vi "测试条件.vi"(11 "TimingControl 输入":refnum<class "TimingControl.lvclass">) -> (2 "簇":cluster{bool, "控制命令":T1, "测量参数":T2}, 3 "TimingControl 输出":refnum<class "TimingControl.lvclass">)   [LabVIEW 2022 SP3, in "TimingControl.lvlib" / "TimingControl.lvclass"]
uses:
  TimingControl.lvclass
  TimingControl.lvclass/TimingControl.ctl
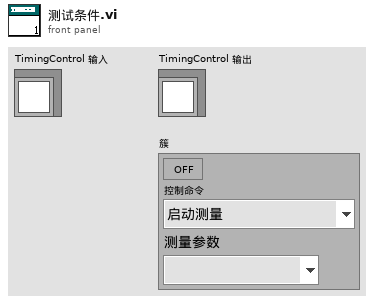
[diagram p1: front panel]
types:
  T1 = typedef "TimingControl.lvlib/TimingControl.lvclass/国标控制命令.ctl" = enum16{"启动测量", "标样核查", "零点核查", "跨度核查", "空白测试", "平行样测试", "加标回收", "空白校准", "标样校准", "初始化（清洗）", "停止测试", "仪器重启", "校时", "模式设置", "测量间隔设置"}
  T2 = typedef "TimingControl.lvlib/TimingControl.lvclass/测量参数.ctl" = u16
  T3 = typedef "TimingControl.lvlib/TimingControl.lvclass/周期模式设置.ctl" = enum16{"不启用", "定点模式", "间隔模式"}
  T4 = typedef "TimingControl.lvlib/TimingControl.lvclass/State Data.ctl" = cluster{"仪器时间":timestamp, "仪器运行状态":bool, "配置文件路径":path, "测量参数":u16, "测试状态":cluster{"启动时间":timestamp, "结束时间":timestamp, "启动次数":i32}, "配置信息":T5}
  T5 = typedef "TimingControl.lvlib/TimingControl.lvclass/配置信息.ctl" = cluster{"每周启动":T6, "每月启动":T7, "周期模式":T3, "测量参数":T2, "定点周期":T8, "间隔启动":T10, "配置时间":timestamp}
  T6 = typedef "TimingControl.lvlib/TimingControl.lvclass/每周启动.ctl" = enum16{"关闭", "周日", "周一", "周二", "周三", "周四", "周五", "周六"}
  T7 = typedef "TimingControl.lvlib/TimingControl.lvclass/每月启动.ctl" = enum16{"关闭", "1号", "2号", "3号", "4号", "5号", "6号", "7号", "8号", "9号", "10号", "11号", "12号", "13号", "14号", "15号", "16号", "17号", "18号", "19号", "20号", "21号", "22号", "23号", "24号", "25号", "26号", "27号", "28号", "29号", "30号", "31号"}
  T8 = typedef "TimingControl.lvlib/TimingControl.lvclass/定点周期设置.ctl" = cluster{"启动命令":T9, "启动命令 2":T9, "启动命令 3":T9, "启动命令 4":T9, "启动命令 5":T9, "启动命令 6":T9, "启动命令 7":T9, "启动命令 8":T9, "启动命令 9":T9, "启动命令 10":T9, "启动命令 11":T9, "启动命令 12":T9, "启动命令 13":T9, "启动命令 14":T9, "启动命令 15":T9, "启动命令 16":T9, "启动命令 17":T9, "启动命令 18":T9, "启动命令 19":T9, "启动命令 20":T9, "启动命令 21":T9, "启动命令 22":T9, "启动命令 23":T9, "启动命令 24":T9}
  T9 = typedef "TimingControl.lvlib/TimingControl.lvclass/启动命令选择.ctl" = enum16{"", "水样测试", "标样核查", "零点核查", "跨度核查", "空白测试", "平行样测试", "加标回收", "空白校准", "标样校准", "初始化(清洗)"}
  T10 = typedef "TimingControl.lvlib/TimingControl.lvclass/间隔启动设置.ctl" = cluster{"启动命令":T9, "启动间隔":dbl, "启动次数":i32}
  T11 = typedef "LVDateTimeRec.ctl" = cluster{"秒数的小数部分":dbl, "秒":i32, "分":i32, "时":i32, "日":i32, "月":i32, "年":i32, "天数（周）":i32, "天数（年）":i32, "DST":i32}
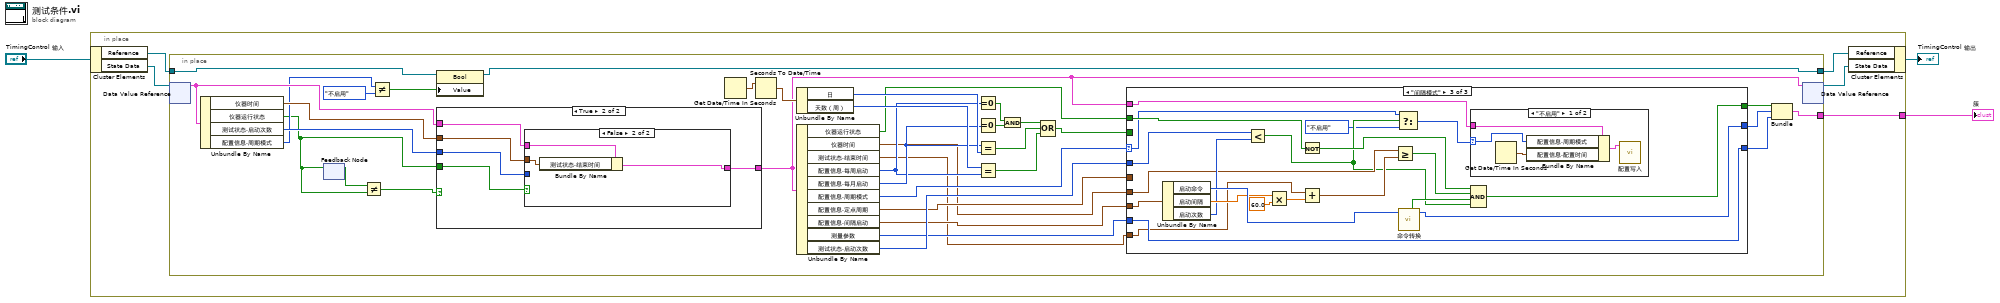
[diagram p0: block diagram]
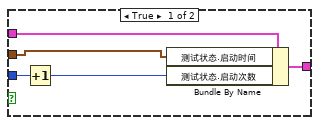
[diagram p3: hidden frame]
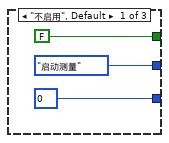
[diagram p4: hidden frame]
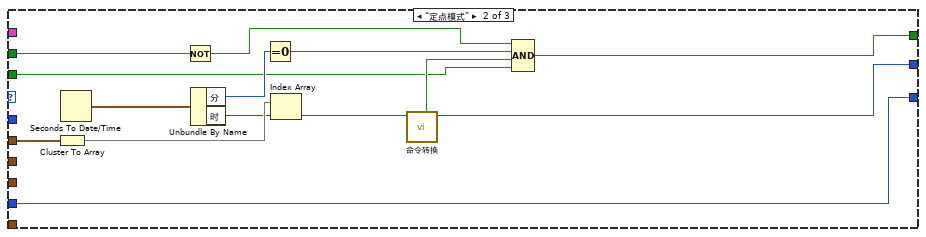
[diagram p5: hidden frame]
diagram:
  n1 = in-place {
    in-place-border: [w8] -> w3
    n2 = in-place-cluster #1("TimingControl 输入") -> ("Reference"=w7:refnum<vi>, "State Data"=w6:refnum<data-value>)
    n3 = in-place {
      in-place-border: w7 -> [w16]
      in-place-border: [w14] -> w8
      in-place-border: [w12] -> w4
      n4 = in-place-dvr #2(w6) -> (w19:T4)  [unwired: 1 out]
      n5 = Unbundle By Name(w19) -> ("仪器时间"=w26:timestamp, "仪器运行状态"=w10:bool, "测试状态.启动次数"=w25:i32, "配置信息.周期模式"=w15:T3)
      n6 = feedback-in #3(w10) -> ()
      n7 = feedback #3() -> (w11:bool)  [unwired: 1 in]
      n8 = Not Equal?(x=w11, y=w10) -> (x != y?=w9:bool)
      n9 = Not Equal?(x=w15, y=周期模式设置."不启用") -> (x != y?=w17:bool)
      n10 = property class="Bool"(reference=w16, "Value"=w17) -> (reference out=w12:refnum<vi>)  [unwired: 1 in, 1 out]
      n11 = case shown="True" w9 {
        tunnel: w26 -> [_ w50]
        tunnel: w25 -> [_ w49]
        tunnel: [w45 w48] -> w13
        tunnel: w19 -> [w45 w47]
        tunnel: w10 -> [_ w46]
        frame False {
        }
        frame True {
          n12 = case shown="False" w46 {
            tunnel: w50 -> [w55 w58]
            tunnel: w49 -> [w53 _]
            tunnel: [w52 w57] -> w48
            tunnel: w47 -> [w51 w56]
            frame True {
              n13 = Increment(x=w53) -> (x+1=w54:i32)
              n14 = Bundle By Name(cluster=w51, "测试状态.启动时间"=w55, "测试状态.启动次数"=w54) -> (w52:T4)
            }
            frame False {
              n15 = Bundle By Name(cluster=w56, "测试状态.结束时间"=w58) -> (w57:T4)
            }
          }
        }
      }
      n16 = Get Date/Time In Seconds() -> (seconds since 1Jan1904=w32:timestamp)
      n17 = Seconds To Date/Time(time stamp (now)=w32) -> (date time rec=w36:T11)  [unwired: 1 in]
      n18 = Unbundle By Name(w36) -> ("日"=w31:i32, "天数（周）"=w35:i32)
      n19 = Unbundle By Name(w13) -> ("仪器运行状态"=w24:bool, "仪器时间"=w21:timestamp, "测试状态.结束时间"=w20:timestamp, "配置信息.每周启动"=w28:T6, "配置信息.每月启动"=w30:T7, "配置信息.周期模式"=w43:T3, "配置信息.定点周期"=w42:T8, "配置信息.间隔启动"=w41:T10, "测量参数"=w40:u16, "测试状态.启动次数"=w44:i32)
      n20 = Equal To 0?(x=w28) -> (x = 0?=w22:bool)
      n21 = Equal To 0?(x=w30) -> (x = 0?=w29:bool)
      n22 = Equal?(x=w30, y=w31) -> (x = y?=w34:bool)
      n23 = Equal?(x=w35, y=w28) -> (x = y?=w33:bool)
      n24 = And(x=w22, y=w29) -> (x .and. y?=w23:bool)
      n25 = Compound Arithmetic op=OR ("复合运算")(w23, w34, w33) -> (w27:bool)
      n26 = case shown="\"间隔模式\"" w43 {
        selector: w43 -> [_ _ w79]
        tunnel: w42 -> [_ w66 _]
        tunnel: w41 -> [_ _ w91]
        tunnel: w40 -> [_ w70 w94]
        tunnel: [国标控制命令."启动测量" ("控制命令") w68 w92] -> w38
        tunnel: [FALSE w71 w95] -> w39
        tunnel: [w59 w70 w94] -> w37
        tunnel: w27 -> [_ w67 _]
        tunnel: w24 -> [_ w62 w84]
        tunnel: w44 -> [_ _ w83]
        tunnel: w20 -> [_ _ w82]
        tunnel: w21 -> [_ _ w81]
        tunnel: w13 -> [_ _ w76]
        frame "不启用", Default {
          w59 = T2 0 items=[""] ("测量参数")
        }
        frame "定点模式" {
          n27 = Cluster To Array(cluster=w66) -> (array=w65:T9[])
          n28 = Seconds To Date/Time() -> (date time rec=w75:T11)  [unwired: 2 in]
          n29 = Not(x=w62) -> (.not. x?=w73:bool)
          n30 = Unbundle By Name(w75) -> ("分"=w74:i32, "时"=w64:i32)
          n31 = Equal To 0?(x=w74) -> (x = 0?=w72:bool)
          n32 = Index Array(array=w65, index=w64) -> (element=w63:T9)
          n33 = call "命令转换.vi"("启动命令"=w63) -> ("控制命令"=w68:T1, "布尔"=w69:bool)  [unwired: 9 in]
          n34 = Compound Arithmetic op=AND ("复合运算")(w73, w72, w69, w67) -> (w71:bool)
        }
        frame "间隔模式" {
          n35 = Unbundle By Name(w91) -> ("启动命令"=w96:T9, "启动间隔"=w90:dbl, "启动次数"=w85:i32)
          n36 = Less?(x=w83, y=w85) -> (x < y?=w80:bool)
          n37 = Multiply(x=w90, y=60.0) -> (x*y=w88:dbl)
          n38 = Not(x=w84) -> (.not. x?=w97:bool)
          n39 = Add(x=w82, y=w88) -> (x+y=w87:timestamp)
          n40 = Greater Or Equal?(x=w81, y=w87) -> (x >= y?=w86:bool)
          n41 = Select(t=w79, s=w80, f=周期模式设置."不启用") -> (s? t:f=w77:T3)
          n42 = call "命令转换.vi"("启动命令"=w96) -> ("控制命令"=w92:T1, "布尔"=w93:bool)  [unwired: 9 in]
          n43 = case shown="\"不启用\"" w77 {
            selector: w77 -> [w99 _]
            tunnel: w76 -> [w101 _]
            frame "不启用" {
              n44 = Get Date/Time In Seconds() -> (seconds since 1Jan1904=w98:timestamp)
              n45 = Bundle By Name(cluster=w101, "配置信息.周期模式"=w99, "配置信息.配置时间"=w98) -> (w100:T4)
              n46 = call "配置写入.vi"("数据值"=w100) -> ()  [unwired: 10 in, 1 out]
            }
            frame "定点模式", Default {
            }
          }
          n47 = Compound Arithmetic op=AND ("复合运算")(w97, w86, w93, w80) -> (w95:bool)
        }
      }
      n48 = Bundle(w39, "控制命令"=w38, "测量参数"=w37) -> (w14:cluster{bool, "控制命令":T1, "测量参数":T2})  [unwired: 1 in]
      n49 = in-place-dvr #2(w13) -> (w5:refnum<data-value>)  [unwired: 1 out]
    }
    n50 = in-place-cluster #1("Reference"=w4, "State Data"=w5) -> (→"TimingControl 输出":refnum<class "TimingControl.lvclass">)
  }
  "簇" <- w3
